vi "open_roller.vi"   [LabVIEW 2013]
uses:
  <vilib>/Rock Robotics/WPI/CAN/Jaguar/SubVIs/WPI_CANJaguar_ControlMode.ctl
  <vilib>/Rock Robotics/WPI/CAN/Jaguar/SubVIs/WPI_CANJaguar_BrakeCoastMode.ctl
  <vilib>/Rock Robotics/WPI/Solenoid/WPI_SolenoidChannel.ctl
  <vilib>/Rock Robotics/SystemInterfaces/Typedef/FPGA_TypedefSolenoidModule.ctl
  <vilib>/Rock Robotics/WPI/Solenoid/WPI_SolenoidValue.ctl
  <vilib>/Rock Robotics/WPI/MotorControl/WPI_MotorControlOpenCANJaguar.vi
  <vilib>/Rock Robotics/WPI/Solenoid/WPI_SolenoidOpenDouble.vi
  <vilib>/Rock Robotics/WPI/Solenoid/WPI_SolenoidSetEnum.vi
types:
  T1 = typedef "WPI_SolenoidValue.ctl" = enum16{"Off", "On", "Forward", "Reverse"}
  T2 = typedef "WPI_SolenoidChannel.ctl" = enum8{"Solenoid 1", "Solenoid 2", "Solenoid 3", "Solenoid 4", "Solenoid 5", "Solenoid 6", "Solenoid 7", "Solenoid 8", "Invalid"}
  T3 = typedef "FPGA_TypedefSolenoidModule.ctl" = enum16{"Solenoid Module 1", "Solenoid Module 2"}
  T4 = typedef "WPI_CANJaguar_BrakeCoastMode.ctl" = enum8{"Jumper", "Brake", "Coast"}
  T5 = typedef "WPI_CANJaguar_ControlMode.ctl" = enum8{"Percent VBus", "Current", "Speed", "Position", "Voltage"}
  T6 = typedef "WPI_MotorControlDeviceRef.ctl" = cluster{"DeviceStatus":errorcluster, "Type":enum16{"PWM", "CAN"}, "PWM":cluster{"Digital Module":T7, "PWM Channel":T8, "DeadBand":T9}, "CAN":cluster{"Device Number":u8, "Control Mode":T5, "Semaphore":T10, "Max Vout":dbl}, "Invert":bool, "TransformRef":T11, "InvTransformRef":T11}
  T7 = typedef "FPGA_TypedefDigitalModule.ctl" = enum16{"Digital Module 1", "Digital Module 2"}
  T8 = typedef "FPGA_DIOPWMChannel.ctl" = enum8{"PWM 1", "PWM 2", "PWM 3", "PWM 4", "PWM 5", "PWM 6", "PWM 7", "PWM 8", "PWM 9", "PWM 10", "Invalid"}
  T9 = typedef "WPI_PWMDeadband.ctl" = cluster{"Name":string, "maxPositivePwm":i32, "minPositivePwm":i32, "centerPwm":i32, "maxNegativePwm":i32, "minNegativePwm":i32, "angularRange":u16}
  T10 = typedef "Semaphore RefNum" = refnum<k1>
  T11 = typedef "WPI_PWMTransform_ConPane.ctl" = refnum<vi>
  T12 = typedef "WPI_SolenoidDevRef.ctl" = cluster{"DevStatus":errorcluster, "Solenoid Module":T3, "Forward Solenoid Channel":T2, "Reverse Solenoid Channel":T2}
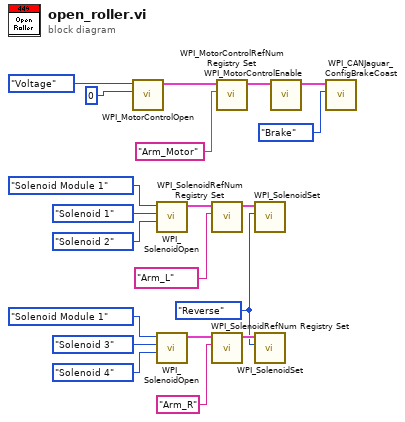
[diagram p0: block diagram]
diagram:
  w1 = WPI_SolenoidValue."Reverse" ("Value")
  n1 = call-poly <vilib>:"WPI_MotorControlOpen.vi"("Device Number"=u8 0, "Control Mode"=WPI_CANJaguar_ControlMode."Voltage") -> ("MotorControlDeviceRef"=w18:T6)  [unwired: 8 in, 1 out]
  n2 = call-poly <vilib>:"WPI_SolenoidOpen.vi"("Reverse Solenoid Channel"=WPI_SolenoidChannel."Solenoid 2", "Forward Solenoid Channel"=WPI_SolenoidChannel."Solenoid 1", "Solenoid Module (Module 1)"=FPGA_TypedefSolenoidModule."Solenoid Module 1") -> ("SolenoidDevRef"=w11:T12)  [unwired: 7 in, 1 out]
  n3 = call-poly <vilib>:"WPI_SolenoidOpen.vi"("Reverse Solenoid Channel"=WPI_SolenoidChannel."Solenoid 4", "Forward Solenoid Channel"=WPI_SolenoidChannel."Solenoid 3", "Solenoid Module (Module 1)"=FPGA_TypedefSolenoidModule."Solenoid Module 1") -> ("SolenoidDevRef"=w7:T12)  [unwired: 7 in, 1 out]
  n4 = call <vilib>:"WPI_SolenoidRefNum Registry Set.vi"("refnum name"="Arm_L", "SolenoidDevRef"=w11) -> ("SolenoidDevRef"=w3:T12)  [unwired: 8 in, 1 out]
  n5 = call <vilib>:"WPI_SolenoidRefNum Registry Set.vi"("refnum name"="Arm_R", "SolenoidDevRef"=w7) -> ("SolenoidDevRef"=w2:T12)  [unwired: 8 in, 1 out]
  n6 = call <vilib>:"WPI_MotorControlRefNum Registry Set.vi"("refnum name"="Arm_Motor", "MotorControlDevRef"=w18) -> ("MotorControlDevRef"=w16:T6)  [unwired: 8 in, 1 out]
  n7 = call-poly <vilib>:"WPI_SolenoidSet.vi"("Value"=w1, "SolenoidDevRef"=w3) -> ()  [unwired: 8 in, 2 out]
  n8 = call-poly <vilib>:"WPI_SolenoidSet.vi"("Value"=w1, "SolenoidDevRef"=w2) -> ()  [unwired: 8 in, 2 out]
  n9 = call <vilib>:"WPI_MotorControlEnable.vi"("CAN Jaguar Ref"=w16) -> ("CAN Jaguar Ref Out"=w15:T6)  [unwired: 9 in, 1 out]
  n10 = call <vilib>:"WPI_CANJaguar_ConfigBrakeCoast.vi"("Brake / Coast Mode"=WPI_CANJaguar_BrakeCoastMode."Brake", "CAN Jaguar Ref"=w15) -> ()  [unwired: 8 in, 2 out]
